vi "Format_DTU.vi"() -> (2 "DTU2":string[](array[string]), 3 "DTU1":string[](array[string]))   [LabVIEW 2024, in "Keyence_VS150.lvlib"]
uses:
  Keyence_VS150.lvlib
  <userlib>/_OpenG.lib/string/string.llb/openg_string.lvlib
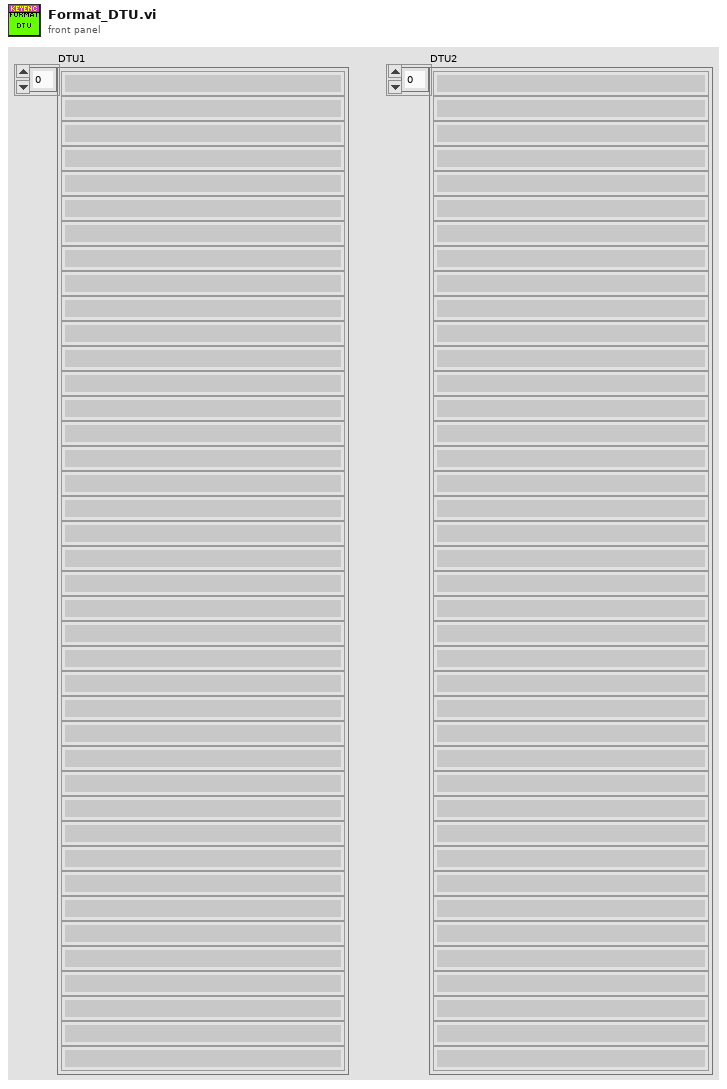
[diagram p1: front panel]
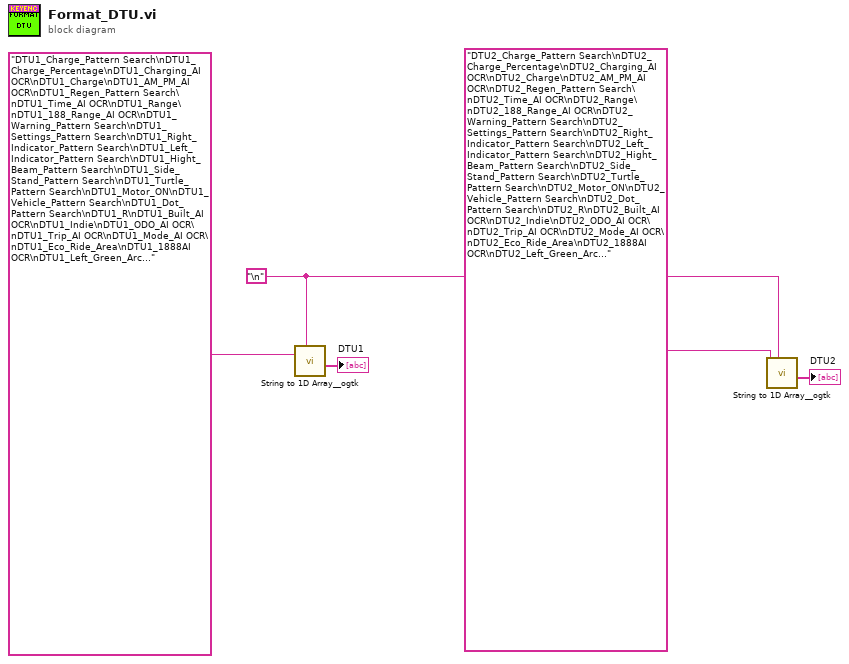
[diagram p0: block diagram]
diagram:
  w2 = "\n"
  n1 = call <userlib>:"String to 1D Array__ogtk.vi"("delimiter (Tab)"=w2, "string"="DTU1_Charge_Pattern Search\nDTU1_Charge_Percentage\nDTU1_Charging_AI OCR\nDTU1_Charge\nDTU1_AM_PM_AI OCR\nDTU1_Regen_Pattern Search\nDTU1_Time_AI OCR\nDTU1_Range\nDTU1_188_Range_AI OCR\nDTU1_Warning_Pattern Search\nDTU1_Settings_Pattern Search\nDTU1_Right_Indicator_Pattern Search\nDTU1_Left_Indicator_Pattern Search\nDTU1_Hight_Beam_Pattern Search\nDTU1_Side_Stand_Pattern Search\nDTU1_Turtle_Pattern Search\nDTU1_Motor_ON\nDTU1_Vehicle_Pattern Search\nDTU1_Dot_Pattern Search\nDTU1_R\nDTU1_Built_AI OCR\nDTU1_Indie\nDTU1_ODO_AI OCR\nDTU1_Trip_AI OCR\nDTU1_Mode_AI OCR\nDTU1_Eco_Ride_Area\nDTU1_1888AI OCR\nDTU1_Left_Green_Arcs_Area\nDTU1_Left_Orange_Area\nDTU1_Left_Violet_Area\nDTU1_Efficiency_AI OCR\nDTU1_Right_Orange_Area\nDTU1_Right_Green_Area\nDTU1_Right_Violet_Area\nDTU1_Warning\nDTU1_Sleep_Mode\nDTU1_km/h_AI OCR\nDTU1_Brake+Start\nDTU1_Segment_Detection\nDTU1_White_Area" ("string (\"\")")) -> ("Array of Strings"=→"DTU1":string[])  [unwired: 9 in]
  n2 = call <userlib>:"String to 1D Array__ogtk.vi"("delimiter (Tab)"=w2, "string"="DTU2_Charge_Pattern Search\nDTU2_Charge_Percentage\nDTU2_Charging_AI OCR\nDTU2_Charge\nDTU2_AM_PM_AI OCR\nDTU2_Regen_Pattern Search\nDTU2_Time_AI OCR\nDTU2_Range\nDTU2_188_Range_AI OCR\nDTU2_Warning_Pattern Search\nDTU2_Settings_Pattern Search\nDTU2_Right_Indicator_Pattern Search\nDTU2_Left_Indicator_Pattern Search\nDTU2_Hight_Beam_Pattern Search\nDTU2_Side_Stand_Pattern Search\nDTU2_Turtle_Pattern Search\nDTU2_Motor_ON\nDTU2_Vehicle_Pattern Search\nDTU2_Dot_Pattern Search\nDTU2_R\nDTU2_Built_AI OCR\nDTU2_Indie\nDTU2_ODO_AI OCR\nDTU2_Trip_AI OCR\nDTU2_Mode_AI OCR\nDTU2_Eco_Ride_Area\nDTU2_1888AI OCR\nDTU2_Left_Green_Arcs_Area\nDTU2_Left_Orange_Area\nDTU2_Left_Violet_Area\nDTU2_Efficiency_AI OCR\nDTU2_Right_Orange_Area\nDTU2_Right_Green_Area\nDTU2_Right_Violet_Area\nDTU2_Warning\nDTU2_Sleep_Mode\nDTU2_km/h_AI OCR\nDTU2_Brake+Start\nDTU2_Segment_Detection\nDTU2_White_Area") -> ("Array of Strings"=→"DTU2":string[])  [unwired: 9 in]
